vi "dd1.vi"(8 "error in":errorcluster, 11 "Class 1 in":refnum<class "Class 1.lvclass">) -> (0 "error out":errorcluster, 3 "Class 1 out":refnum<class "Class 1.lvclass">)   [LabVIEW 2026, in "Class 1.lvclass"]
uses:
  Class 1.lvclass
  Class 1.lvclass/Class 1.ctl
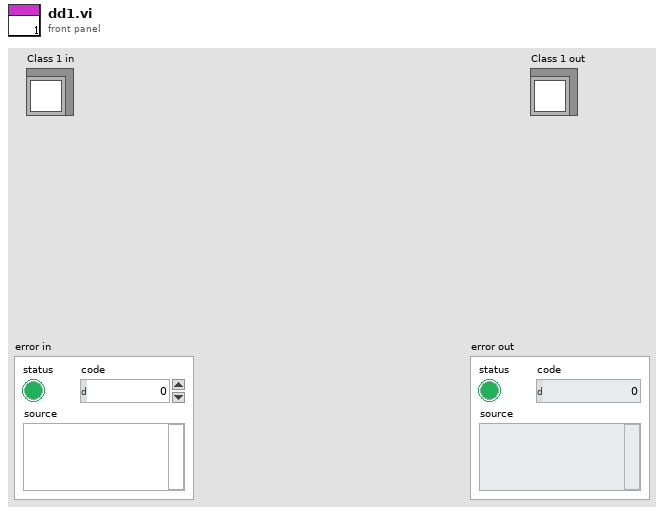
[diagram p1: front panel]
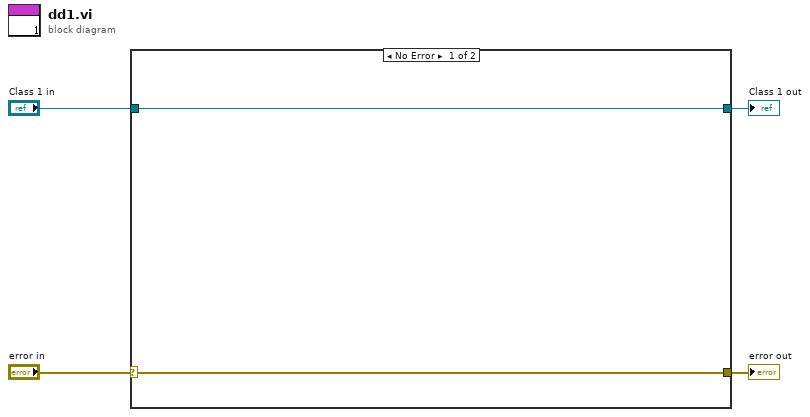
[diagram p0: block diagram]
diagram:
  n1 = case shown="No Error" "error in" {
    selector: "error in" -> [w5 w8]
    tunnel: [w5 w8] -> w1
    tunnel: [w6 w7] -> w3
    tunnel: "Class 1 in" -> [w6 w7]
    frame No Error {
    }
    frame Error {
    }
  }
  "Class 1 out" <- w3
  "error out" <- w1
